vi "Init AWG.vi"(8 "error in (no error)":errorcluster, 11 "QPS settings":T21 {"awg"."HMF2500 cfg"."Flow Control" items=["None", "XON/XOFF", "RTS/CTS", "XON/XOFF & RTS/CTS", "DTR/DSR", "XON/XOFF & DTR/DSR"]; "awg"."HMF2500 cfg"."Data Bits" items=["7"=7, "8"=8]; "awg"."HMF2500 cfg"."Parity" items=["None", "Odd", "Even", "Mark", "Space"]; "awg"."HMF2500 cfg"."Baud Rate" items=["300"=300, "600"=600, "1200"=1200, "2400"=2400, "4800"=4800, "9600"=9600, "19200"=19200]; "awg"."cmi sync v3"."chn2 div" min=1 max=100000000 step=1; "awg"."cmi sync v3"."fsrc [Hz]" format="%_8p"; "PJVS setup"."NPL bias source"."DataSocketCluster"."TimeStamp" format="%.2f"; "meas"."Calculated"."Trigger frequency  (Hz)" format="%#_6p"; "meas"."Record length (multiples of M)" min=1 step=1; "meas"."PJVS reference voltages (1 period, V)" format="%.9g"; "meas"."MRe (s)" format="%#_4p"; "meas"."MRs (s)" format="%#_4p"; "meas"."PRe (s)" format="%#.4p"; "meas"."PRs (s)" format="%#_4p"}) -> (0 "error out":errorcluster, 3 "awg session out":T2 {"HMF2500 cfg"."Flow Control" items=["None", "XON/XOFF", "RTS/CTS", "XON/XOFF & RTS/CTS", "DTR/DSR", "XON/XOFF & DTR/DSR"]; "HMF2500 cfg"."Data Bits" items=["7"=7, "8"=8]; "HMF2500 cfg"."Parity" items=["None", "Odd", "Even", "Mark", "Space"]; "HMF2500 cfg"."Baud Rate" items=["300"=300, "600"=600, "1200"=1200, "2400"=2400, "4800"=4800, "9600"=9600, "19200"=19200]; "cmi sync v3"."chn2 div" min=1 max=100000000 step=1; "cmi sync v3"."fsrc [Hz]" format="%_8p"})   [LabVIEW 2020]
uses:
  external libraries/AWG/AWG.lvlib
  external libraries/AWG/AWG Clock Setup Mode.ctl
  external libraries/externals needed for AWG/3458A Sampling Rate.ctl
  external libraries/externals needed for AWG/ADC Trig Slope.ctl
  external libraries/externals needed for AWG/ADC Trig Coupling.ctl
  external libraries/externals needed for AWG/ADC Trig Mode Source.ctl
  external libraries/externals needed for AWG/ADC Trig Config.ctl
  Measurement/Type definitions/Measurement ID.ctl
  Measurement/Type definitions/Trigger mode.ctl
  Measurement/Type definitions/Measuement properties.ctl
  General PJVS driver/Type definitions/PJVS Type.ctl
  PJVS drivers/acsvcontrol-driver/build/ACSVcontrol-driver_0.2.0.0.llb/Timeouts.ctl
  PJVS drivers/acsvcontrol-driver/build/ACSVcontrol-driver_0.2.0.0.llb/ACSVcontrol-driver.lvlib
  PJVS drivers/JV modified NPL Bias source/DataSocketCluster external.ctl
  General PJVS driver/Type definitions/PJVS Setup.ctl
  external libraries/AWG/AWG Type.ctl
  external libraries/AWG/CMI Clock Divider v2/CMI ckd2 Source Mode.ctl
  external libraries/AWG/CMI Clock Divider v2/CMI ckd2 Divisor Mode.ctl
  external libraries/AWG/CMI Clock Divider v2/CMI ckd2 Session.ctl
  external libraries/AWG/CMI Sync V3/Configure/CMI Sync V3 Reference Clock Source.ctl
  external libraries/AWG/CMI Sync V3/CMI Sync Unit V3.lvlib
  external libraries/AWG/CMI Sync V3/Configure/CMI Sync V3 HV input Range.ctl
  external libraries/AWG/CMI Sync V3/Configure/CMI Sync V3 Trigger Input Level.ctl
  external libraries/AWG/CMI Sync V3/Configure/CMI Sync V3 Channel 1 Mode.ctl
  external libraries/AWG/CMI Sync V3/Configure/CMI Sync V3 Channel Output Levels.ctl
  external libraries/AWG/CMI Sync V3/Configure/CMI Sync V3 Channel 2 Mode.ctl
  external libraries/AWG/CMI Sync V3/Configure/CMI Sync V3 Channel 3 Mode.ctl
  external libraries/AWG/CMI Sync V3/Configure/CMI Sync V3 Channel 1 Divisor Entry Mode.ctl
  external libraries/AWG/CMI Sync V3/CMI Sync V3 session.ctl
  external libraries/AWG/RaS HMF2500/HMF2500 Config.ctl
  external libraries/AWG/AWG Session.ctl
  General PJVS driver/QPSsettings.ctl
  Type definitions/AWG type.ctl
panel:
  in  "AWG type":T1
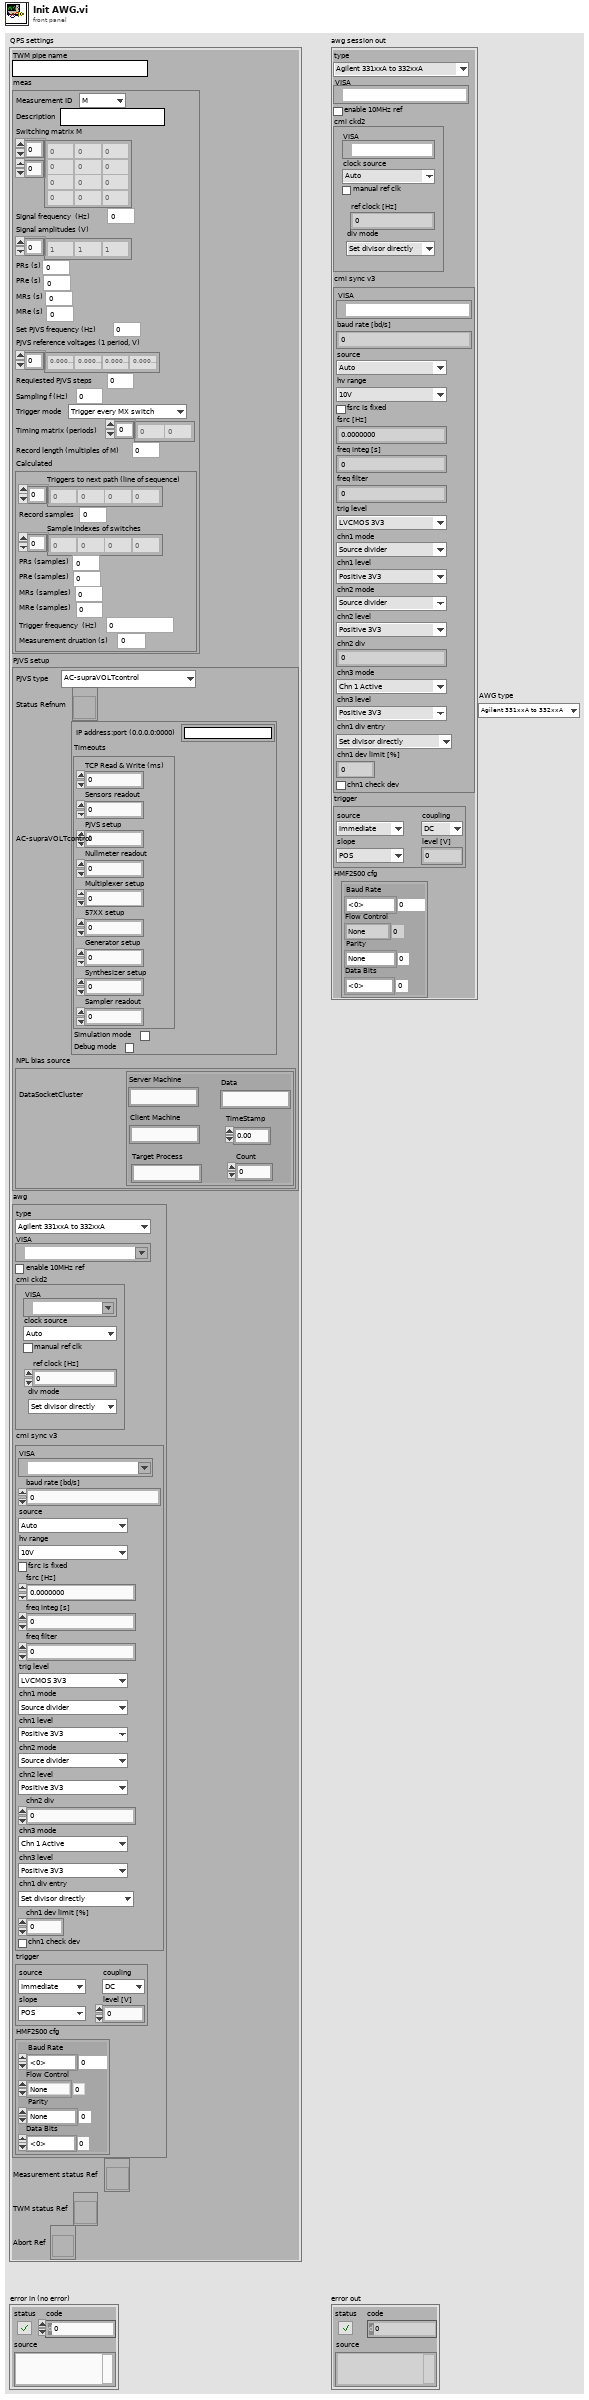
[diagram p1: front panel]
types:
  T1 = typedef "AWG type.ctl" = enum16{"Agilent 331xxA to 332xxA", "Agilent 335xxA to 336xxA", "Tektronix AFG3101C", "R&S HMF25xx", "CMI Clock Divider v2", "CMI Sync Unit V3", "FGEN NI 5413", "Supracon PJVS Generator", "dummy"}
  T2 = typedef "AWG.lvlib/AWG Session.ctl" = cluster{"type":T3, "VISA":refnum<visa-resource-name>, "enable 10MHz ref":bool, "cmi ckd2":T4, "cmi sync v3":T7, "trigger":T16, "HMF2500 cfg":T20}
  T3 = typedef "AWG.lvlib/AWG Type.ctl" = enum16{"Agilent 331xxA to 332xxA", "Agilent 335xxA to 336xxA", "Tektronix AFG3101C", "R&S HMF25xx", "CMI Clock Divider v2", "CMI Sync Unit V3", "dummy"}
  T4 = typedef "AWG.lvlib/CMI ckd2 Session.ctl" = cluster{"VISA":refnum<visa-resource-name>, "clock source":T5, "manual ref clk":bool, "ref clock [Hz]":dbl, "div mode":T6}
  T5 = typedef "AWG.lvlib/CMI ckd2 Source Mode.ctl" = enum16{"Auto", "LF clock", "HF clock", "Internal"}
  T6 = typedef "AWG.lvlib/CMI ckd2 Divisor Mode.ctl" = enum16{"Set divisor directly", "Set divisor by frequency"}
  T7 = typedef "AWG.lvlib/CMI Sync Unit V3.lvlib/CMI Sync V3 session.ctl" = cluster{"VISA":refnum<visa-resource-name>, "baud rate [bd/s]":i32, "source":T8, "hv range":T9, "fsrc is fixed":bool, "fsrc [Hz]":dbl, "freq integ [s]":dbl, "freq filter":i32, "trig level":T10, "chn1 mode":T11, "chn1 level":T12, "chn2 mode":T13, "chn2 level":T12, "chn2 div":i32, "chn3 mode":T14, "chn3 level":T12, "chn1 div entry":T15, "chn1 dev limit [%]":dbl, "chn1 check dev":bool}
  T8 = typedef "AWG.lvlib/CMI Sync Unit V3.lvlib/CMI Sync V3 Reference Clock Source.ctl" = enum16{"Auto", "Internal", "Logic", "Sine", "HV"}
  T9 = typedef "AWG.lvlib/CMI Sync Unit V3.lvlib/CMI Sync V3 HV input Range.ctl" = enum16{"10V", "60V", "250V", "1kV"}
  T10 = typedef "AWG.lvlib/CMI Sync Unit V3.lvlib/CMI Sync V3 Trigger Input Level.ctl" = enum16{"LVCMOS 3V3", "TTL 5V"}
  T11 = typedef "AWG.lvlib/CMI Sync Unit V3.lvlib/CMI Sync V3 Channel 1 Mode.ctl" = enum16{"Source divider", "DDS absolute", "DDS ratio", "DDS ratio M/N"}
  T12 = typedef "AWG.lvlib/CMI Sync Unit V3.lvlib/CMI Sync V3 Channel Output Levels.ctl" = enum16{"Positive 3V3", "Negative 3V3", "Positive 5V", "Negative 5V"}
  T13 = typedef "AWG.lvlib/CMI Sync Unit V3.lvlib/CMI Sync V3 Channel 2 Mode.ctl" = enum16{"Source divider", "Chn 1 divide"}
  T14 = typedef "AWG.lvlib/CMI Sync Unit V3.lvlib/CMI Sync V3 Channel 3 Mode.ctl" = enum16{"Chn 1 Active", "Chn 2 Active", "Chn 1 Trigger", "Chn 2 Trigger", "Gate", "PPS", "10MHz"}
  T15 = typedef "AWG.lvlib/CMI Sync Unit V3.lvlib/CMI Sync V3 Channel 1 Divisor Entry Mode.ctl" = enum16{"Set divisor directly", "Calculate nearest divisor from measured fx"}
  T16 = typedef "ADC Trig Config.ctl" = cluster{"source":T17, "level [V]":dbl, "coupling":T18, "slope":T19}
  T17 = typedef "ADC Trig Mode Source.ctl" = enum16{"Immediate", "External", "Level"}
  T18 = typedef "ADC Trig Coupling.ctl" = enum16{"DC", "AC"}
  T19 = typedef "ADC Trig Slope.ctl" = enum16{"POS", "NEG"}
  T20 = typedef "AWG.lvlib/HMF2500 Config.ctl" = cluster{"Baud Rate":u32, "Parity":u16, "Data Bits":u16, "Flow Control":u16}
  T21 = typedef "QPSsettings.ctl" = cluster{"TWM pipe name":string, "meas":T22, "PJVS setup":T25, "awg":T2, "Measurement status Ref":refnum<vi>, "TWM status Ref":refnum<vi>, "Abort Ref":refnum<vi>}
  T22 = typedef "Measuement properties.ctl" = cluster{"Measurement ID":T23, "Description":string, "Switching matrix M":u32[][], "Signal frequency  (Hz)":dbl, "Signal amplitudes (V)":dbl[], "PRs (s)":dbl, "PRe (s)":dbl, "MRs (s)":dbl, "MRe (s)":dbl, "Set PJVS frequency (Hz)":dbl, "PJVS reference voltages (1 period, V)":dbl[], "Requiested PJVS steps":u32, "Sampling f (Hz)":dbl, "Trigger mode":T24, "Timing matrix (periods)":i32[], "Record length (multiples of M)":u32, "Calculated":cluster{"Triggers to next path (line of sequence)":u32[], "Record samples":u32, "Sample indexes of switches":u32[], "PRs (samples)":i32, "PRe (samples)":i32, "MRs (samples)":i32, "MRe (samples)":i32, "Trigger frequency  (Hz)":dbl, "Measurement druation (s)":dbl}}
  T23 = typedef "Measurement ID.ctl" = enum16{"M", "1", "2", "3"}
  T24 = typedef "Trigger mode.ctl" = enum16{"Trigger every MX switch", "Trigger every sample"}
  T25 = typedef "PJVS Setup.ctl" = cluster{"PJVS type":T26, "Status Refnum":refnum<vi>, "AC-supraVOLTcontrol":cluster{"IP address:port (0.0.0.0:0000)":string, "Timeouts":T27, "Simulation mode":bool, "Debug mode":bool}, "NPL bias source":cluster{"DataSocketCluster":T28}}
  T26 = typedef "PJVS Type.ctl" = enum16{"AC-supraVOLTcontrol", "JV modified NPL bias control"}
  T27 = typedef "ACSVcontrol-driver.lvlib/Timeouts.ctl" = cluster{"TCP Read & Write (ms)":i32, "Sensors readout":i32, "PJVS setup":i32, "Nullmeter readout":i32, "Multiplexer setup":i32, "57XX setup":i32, "Generator setup":i32, "Synthesizer setup":i32, "Sampler readout":i32}
  T28 = typedef "DataSocketCluster external.ctl" = cluster{"Server Machine":string, "Client Machine":string, "Data":string, "TimeStamp":dbl, "Count":i32, "Target Process":string}
  T29 = typedef "AWG.lvlib/AWG Clock Setup Mode.ctl" = enum16{"fs or Ts", "fs or Ts with fref", "fref/N", "fref*M/N", "fref*Ratio"}
  T30 = typedef "3458A Sampling Rate.ctl" = cluster{"freq mode":T29, "fs [Hz]":dbl, "fref [Hz]":dbl, "mul":dbl, "div":dbl}
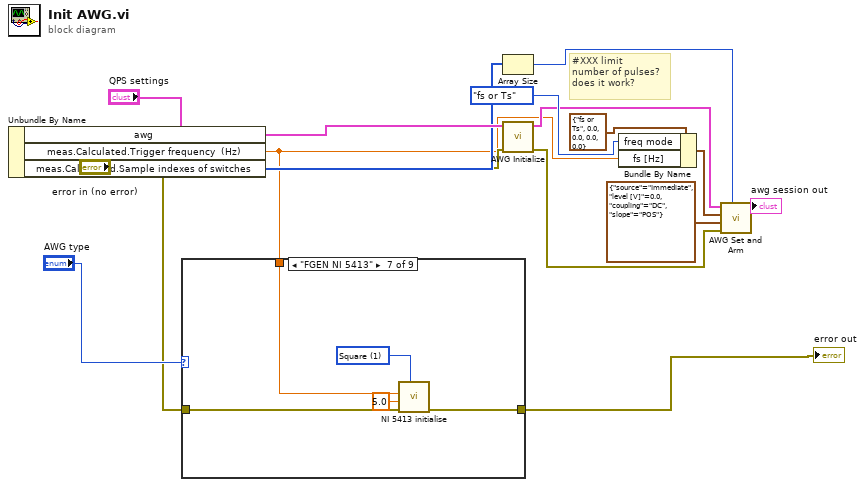
[diagram p0: block diagram]
diagram:
  # "#XXX limit \nnumber of pulses?\ndoes it work?"
  n1 = Unbundle By Name("QPS settings") -> ("awg"=w14:T2, "meas.Calculated.Trigger frequency  (Hz)"=w1:dbl, "meas.Calculated.Sample indexes of switches"=w13:u32[])
  n2 = case shown="\"FGEN NI 5413\"" "AWG type" {
    tunnel: "error in (no error)" -> [_ _ _ _ _ _ w20 _ _]
    tunnel: [_ _ _ _ _ _ w19 _ _] -> w2
    tunnel: w1 -> [_ _ _ _ _ _ w18 _ _]
    frame "Agilent 331xxA to 332xxA", Default {
    }
    frame "Agilent 335xxA to 336xxA" {
    }
    frame "Tektronix AFG3101C" {
    }
    frame "R&S HMF25xx" {
    }
    frame "CMI Clock Divider v2" {
    }
    frame "CMI Sync Unit V3" {
    }
    frame "FGEN NI 5413" {
      w16 = u16 1 items=["Sine", "Square", "Triangle", "Ramp Up", "Ramp Down", "DC", "Noise"] ("Standard Waveform")
      n3 = call "NI 5413 initialise.vi"("Standard Waveform"=w16, "error in (no error)"=w20, "Amplitude"=5.0, "Frequency"=w18) -> ("error out"=w19:errorcluster)  [unwired: 6 in, 1 out]
    }
    frame "Supracon PJVS Generator" {
    }
    frame "dummy" {
    }
  }
  "error out" <- w2
  n4 = Array Size(array=w13) -> (size(s)=w15:i32)
  n5 = call "AWG Initialize.vi"("error in (no error)"="error in (no error)", "awg session in"=w14) -> ("error out"=w5:errorcluster, "awg session out"=w6:T2)  [unwired: 7 in, 1 out]
  n6 = Bundle By Name(cluster=T30 {"freq mode"=enum."fs or Ts", "fs [Hz]"=0.0, "fref [Hz]"=0.0, "mul"=0.0, "div"=0.0} ("sampling rate"), "freq mode"=AWG_Clock_Setup_Mode."fs or Ts", "fs [Hz]"=w1) -> (w10:T30)
  n7 = call "AWG Set and Arm.vi"("pulse count (0: infinite)"=w15, "error in (no error)"=w5, "trigger"=T16 {"source"=enum."Immediate", "level [V]"=0.0, "coupling"=enum."DC", "slope"=enum."POS"}, "sampling rate"=w10, "awg session in"=w6) -> ("awg session out"=→"awg session out":T2)  [unwired: 5 in, 1 out]
